vi "sub_DoubleTone.vi"(6 "Sound Format":T1={"sample rate (S/s)"=22050.0, "number of channels"=1, "bits per sample"=16}, 7 "amplitude":dbl=0.5 format="%#_13g", 8 "error in (no error)":errorcluster, 9 "Play time (sec)":dbl=2.0, 10 "2nd frequency (Hz)":dbl=697.0, 11 "1st frequency (Hz)":dbl=1209.0) -> (0 "error out":errorcluster, 3 "signal out":waveform(dbl), 4 "#s":dbl)   [LabVIEW 2014]
doc: "------------------------------------\nAuther: Koji Ohashi\nCopyright (c) 2020 Japan LabVIEW Users Group, Volunteer members.\nThis VI is released under the MIT License.\nhttp://opensource.org/licenses/mit-license.php\n------------------------------------"
uses:
  <vilib>/measure/NI_MABase.lvlib
  <vilib>/sound2/lvsound2.llb/Sound Data Format.ctl
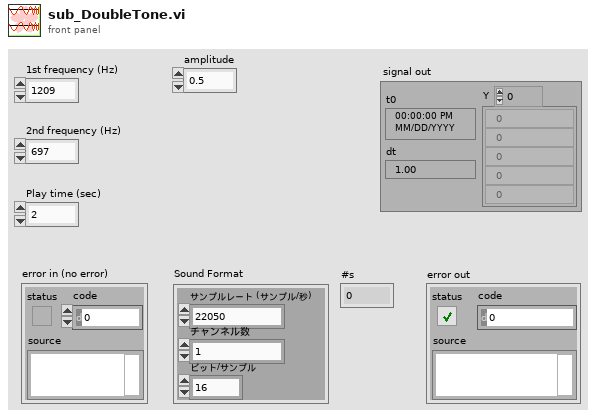
[diagram p1: front panel]
types:
  T1 = typedef "Sound Data Format.ctl" = cluster{"sample rate (S/s)":dbl, "number of channels":i32, "bits per sample":i32}
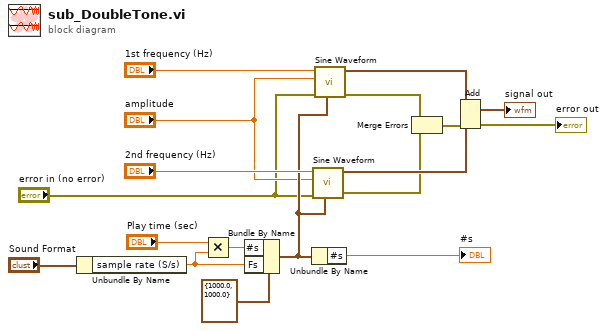
[diagram p0: block diagram]
diagram:
  n1 = Unbundle By Name("Sound Format") -> ("sample rate (S/s)"=w15:dbl)
  n2 = Multiply(x="Play time (sec)", y=w15) -> (x*y=w8:dbl)
  n3 = Bundle By Name(cluster=cluster{"Fs":dbl, "#s":dbl} {"Fs"=1000.0, "#s"=1000.0} ("sampling info"), "#s"=w8, "Fs"=w15) -> (w12:cluster{"Fs":dbl, "#s":dbl})
  n4 = Unbundle By Name(w12) -> ("#s"=→"#s":dbl)
  n5 = call <vilib>:"Sine Waveform.vi"("sampling info"=w12, "error in (no error)"="error in (no error)", "amplitude"="amplitude", "frequency"="2nd frequency (Hz)") -> ("error out"=w3:errorcluster, "signal out"=w10:waveform(dbl))  [unwired: 6 in]
  n6 = call <vilib>:"Sine Waveform.vi"("sampling info"=w12, "error in (no error)"="error in (no error)", "amplitude"="amplitude", "frequency"="1st frequency (Hz)") -> ("error out"=w4:errorcluster, "signal out"=w11:waveform(dbl))  [unwired: 6 in]
  n7 = Merge Errors(w4, w3) -> (w2:errorcluster)
  n8 = Add(1:w10, 2:w11, 4:w2) -> (0:→"signal out":waveform(dbl), 3:→"error out":errorcluster)
